vi "MFLI_File_read.vi"(6 "Type (text)":enum16{"bin", "text"}(ring)=enum."text", 8 "Error In":errorcluster, 9 "access (0:read/write)":enum16{"read/write", "read-only", "write-only"}(ring), 10 "operation (0:open)":T1(ring), 11 "Project script or program":path) -> (0 "Error Out":errorcluster, 3 "String":string)   [LabVIEW 2018]
uses:
  <vilib>/addons/Tools/Unicode/UTF8 Tools.lvlib
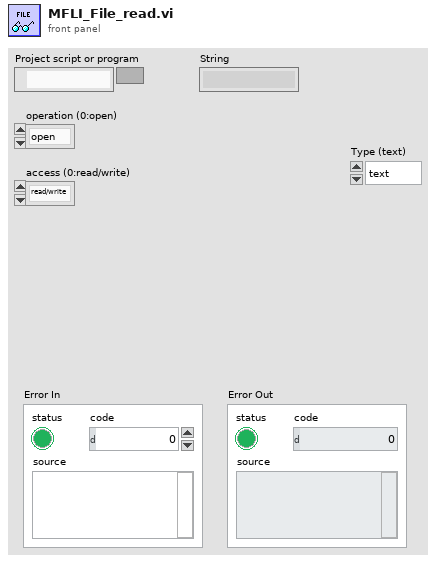
[diagram p1: front panel]
types:
  T1 = enum16{"open", "replace", "create", "open or create", "replace or create", "replace or create with confirmation"}
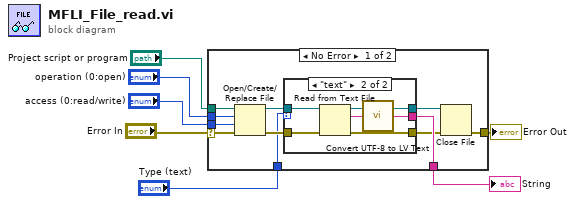
[diagram p0: block diagram]
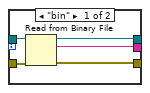
[diagram p2: hidden frame]
diagram:
  n1 = case shown="No Error" "Error In" {
    selector: "Error In" -> [w9 w30]
    tunnel: [w18 w30] -> w1
    tunnel: [w17 _] -> w7
    tunnel: "access (0:read/write)" -> [w16 _]
    tunnel: "operation (0:open)" -> [w15 _]
    tunnel: "Project script or program" -> [w14 _]
    tunnel: "Type (text)" -> [w8 _]
    frame No Error {
      n2 = Open/Create/Replace File(file path (use dialog)=w14, error in=w9, operation (0:open)=w15, access (0:read/write)=w16) -> (refnum out=w13:refnum<file>, error out=w10:errorcluster)  [unwired: 2 in, 1 out]
      n3 = case shown="\"text\"" w8 {
        tunnel: [w19 w24] -> w17
        tunnel: w13 -> [w21 w29]
        tunnel: [w20 w28] -> w12
        tunnel: [w22 w27] -> w11
        tunnel: w10 -> [w23 w26]
        frame "bin" {
          n4 = Read from Binary File(8:w23, 11:w21) -> (0:w22:errorcluster, 2:w19:string, 3:w20:refnum<file>)  [unwired: 4 in, 1 out]
        }
        frame "text" {
          n5 = Read from Text File(file (use dialog)=w29, error in=w26) -> (refnum out=w28:refnum<file>, text=w25:string, error out=w27:errorcluster)  [unwired: 2 in, 1 out]
          n6 = call <vilib>:"Convert UTF-8 to LV Text.vi"("UTF-8 Text"=w25) -> ("LV Text"=w24:string)  [unwired: 13 in, 1 out]
        }
      }
      n7 = Close File(refnum=w12, error in=w11) -> (error out=w18:errorcluster)  [unwired: 1 out]
    }
    frame Error {
    }
  }
  "String" <- w7
  "Error Out" <- w1
